vi "mhk_velmex.vi"() -> ()   [LabVIEW 2010]
panel:
  in  "SEND COMMAND":bool
  out "Command String":string
  in  "Number of Steps":u32(knob)=1 min=1 max=100000 step=1 scale=1.0..100000.0
  in  "Direction":bool
  in  "Motor Speed\n(Steps/sec)":i32(knob)=2000 min=2000 max=8000 scale=2000.0..8000.0
  in  "Motor Number":dbl=1.0 min=1.0 max=4.0 step=1.0
  # "Negative"
  # "Positive"
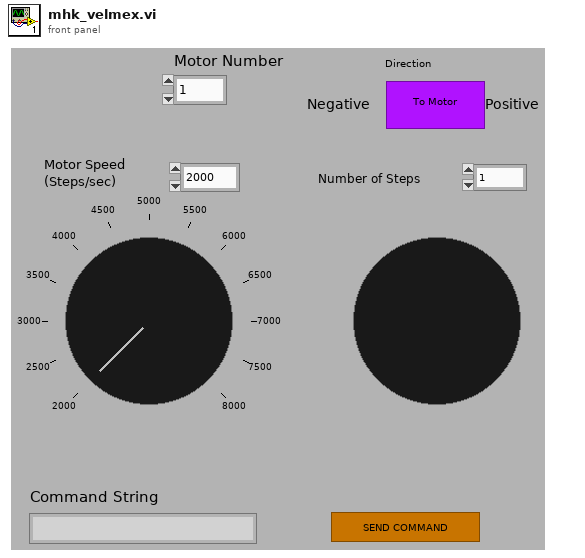
[diagram p1: front panel]
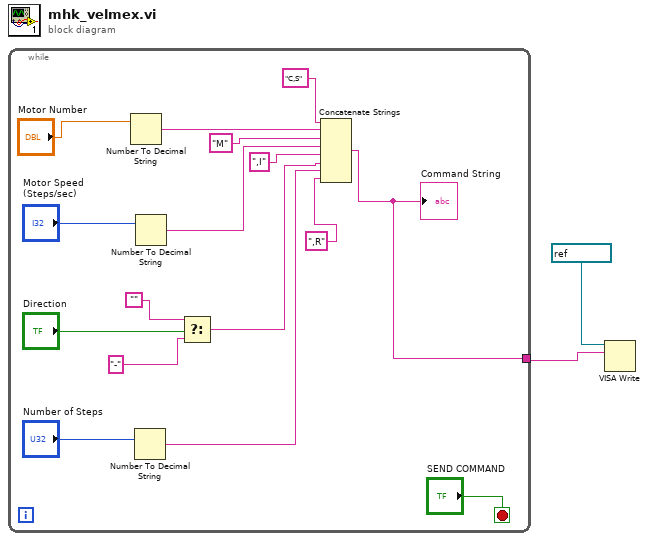
[diagram p0: block diagram]
diagram:
  n1 = while {
    tunnel: [w4] -> w2
    stop <- "SEND COMMAND" stop-if-true
    n2 = Number To Decimal String(number="Motor Number") -> (decimal integer string=w11:string)  [unwired: 1 in]
    n3 = Number To Decimal String(number="Number of Steps") -> (decimal integer string=w6:string)  [unwired: 1 in]
    n4 = Number To Decimal String(number="Motor Speed\n(Steps/sec)") -> (decimal integer string=w9:string)  [unwired: 1 in]
    n5 = Select(t="", s="Direction", f="-") -> (s? t:f=w7:string)
    n6 = Concatenate Strings("C,S", w11, "M", w9, ",I", w7, w6, ",R") -> (w4:string)
    "Command String" <- w4
  }
  n7 = VISA Write(VISA resource name=refnum<visa-resource-name> "COM1", write buffer=w2) -> ()  [unwired: 1 in, 3 out]
